vi "FTWLib-SQLite-LibraryFilepath.vi"(8 "error in":errorcluster) -> (0 "error out":errorcluster, 1 "SQLite Version":string, 2 "SQLite Library Filepath":path)   [LabVIEW 2014]
uses:
  src/core/error/FTW-ERR-ThrowError.vi
  src/core/error/FTW-ERR-NoErrorConstant.vi
  src/core/string/FTW-STR-ReplaceWhitespace.vi
  src/core/error/FTW-ERR-CallChain.vi
  FTWLib-SQLite32.dll
  FTWLib-SQLite64.dll
  FTWLib-SQLite32.so
panel:
  # "Inputs"
  # "Outputs"
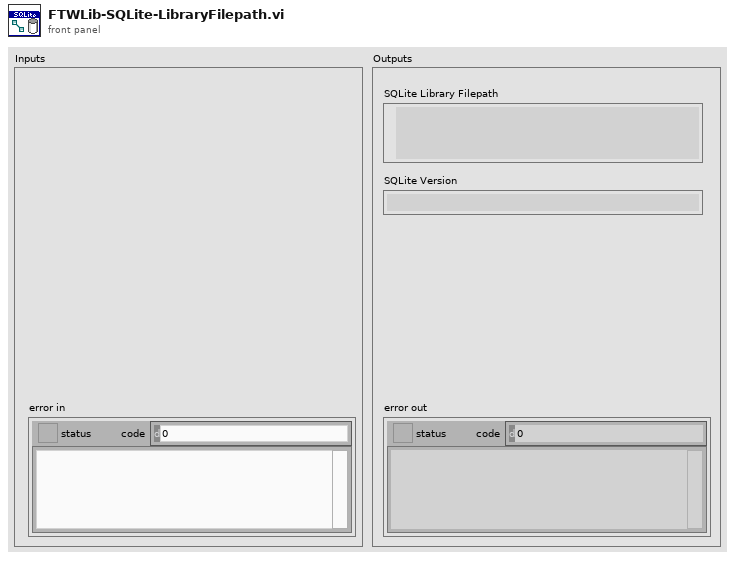
[diagram p1: front panel]
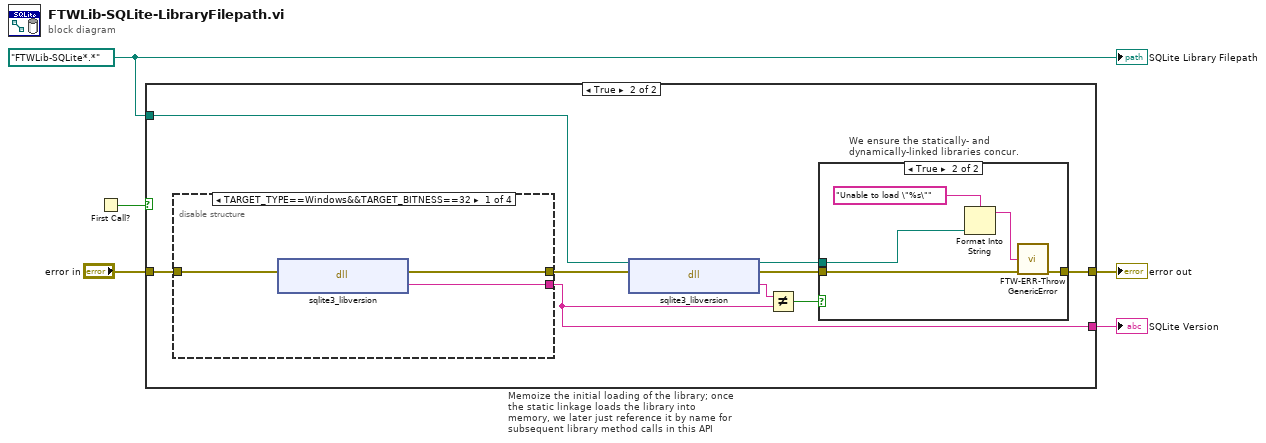
[diagram p0: block diagram]
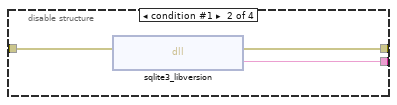
[diagram p4: hidden frame]
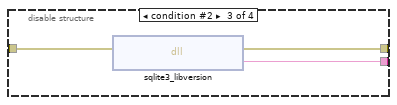
[diagram p5: hidden frame]
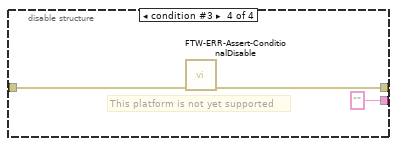
[diagram p6: hidden frame]
diagram:
  w2 = path "FTWLib-SQLite*.*"
  n1 = First Call?() -> (First Call?: T/F=w1:bool)
  n2 = case "Memoize the initial loading of the library; once the static linkage loads the library into memory, we later just reference it by name for subsequent library method calls in this API" shown="True" w1 {
    tunnel: "error in" -> [w6 w15]
    tunnel: [_ w13] -> w3
    tunnel: [w6 w10] -> w4
    tunnel: w2 -> [_ w9]
    frame False {
    }
    frame True {
      n3 = disable-structure shown="TARGET_TYPE==Windows&&TARGET_BITNESS==32" {
        disable-tunnel: [w23 w26 w29 w31] -> w8
        disable-tunnel: w15 -> [w24 w27 w30 w32]
        disable-tunnel: [w22 w25 w28 "" ("Return Value")] -> w13
        frame condition #0 (active) {
          n4 = dll-call lib="C:/Users/Jack/repo/ftw-master/ftw/lib/sqlite/FTWLib-SQLite32.dll" fn="sqlite3_libversion" label="FTWLib-SQLite32.dll"(error in=w24) -> (error out=w23:errorcluster, "Return Value"=w22:string)  [unwired: 2 in, 1 out]
        }
        frame condition #1 {
          n5 = dll-call lib="C:/Users/Jack/repo/ftw-master/ftw/lib/sqlite/FTWLib-SQLite64.dll" fn="sqlite3_libversion" label="FTWLib-SQLite64.dll"(error in=w27) -> (error out=w26:errorcluster, "Return Value"=w25:string)  [unwired: 2 in, 1 out]
        }
        frame condition #2 {
          n6 = dll-call lib="C:/Users/Jack/repo/ftw-master/ftw/lib/sqlite/FTWLib-SQLite32.so" fn="sqlite3_libversion" label="FTWLib-SQLite32.so"(error in=w30) -> (error out=w29:errorcluster, "Return Value"=w28:string)  [unwired: 2 in, 1 out]
        }
        frame condition #3 {
          # "This platform is not yet supported"
          n7 = call "FTW-ERR-Assert-ConditionalDisable.vi"("error in"=w32) -> ("error out"=w31:errorcluster)  [unwired: 14 in]
        }
      }
      n8 = dll-call lib="?" fn="sqlite3_libversion"(path in=w9, error in=w8) -> (path out=w7:path, error out=w11:errorcluster, "Return Value"=w14:string)  [unwired: 1 in]
      n9 = Not Equal?(x=w14, y=w13) -> (x != y?=w12:bool)
      n10 = case "We ensure the statically- and\ndynamically-linked libraries concur." shown="True" w12 {
        tunnel: w11 -> [w16 w21]
        tunnel: [w16 w20] -> w10
        tunnel: w7 -> [_ w19]
        frame False {
        }
        frame True {
          n11 = Format Into String(format string="Unable to load \"%s\"", w19) -> (resulting string=w18:string)  [unwired: 2 in, 1 out]
          n12 = call "FTW-ERR-ThrowGenericError.vi"("Error Message"=w18, "error in"=w21) -> ("error out"=w20:errorcluster)  [unwired: 13 in]
        }
      }
    }
  }
  "error out" <- w4
  "SQLite Version" <- w3
  "SQLite Library Filepath" <- w2
